vi "Test 1 Error Method.vi"(8 "error in (no error)":errorcluster, 11 "Test Test Case in":refnum<class "Error First Test Case.lvclass">) -> (0 "error out":errorcluster, 3 "Test Test Case out":refnum<class "Error First Test Case.lvclass">)   [LabVIEW 2020, in "Error First Test Case.lvclass"]
uses:
  Error First Test Case.lvclass
  source/Framework/Test Case/LUnit Test Case.lvclass
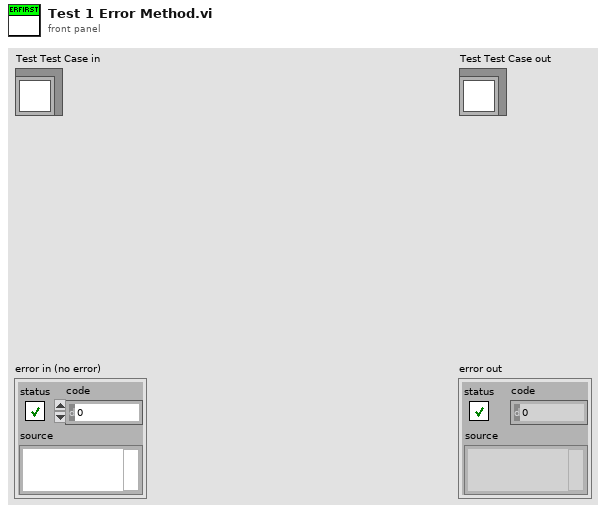
[diagram p1: front panel]
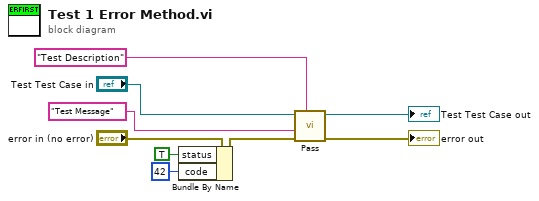
[diagram p0: block diagram]
diagram:
  n1 = Bundle By Name(cluster="error in (no error)", "status"=TRUE, "code"=42) -> (w3:errorcluster)
  n2 = call "Pass.vi"("Description"="Test Description", "error in (no error)"=w3, "Message"="Test Message", "LUnit Test Case In"="Test Test Case in") -> ("error out"=→"error out":errorcluster, "LUnit Test Case Out"=→"Test Test Case out":refnum<class "Error First Test Case.lvclass">)  [unwired: 6 in]
